vi "Measurement.Free.Initialize.vi"(8 "error in (no error)":errorcluster, 9 "timeout (5000 ms)":i32=5000, 11 "Measurement.Free in":refnum<class "Measurement.Free.lvclass">) -> (0 "error out":errorcluster, 1 "Init complete":bool, 3 "Measurement.Free out":refnum<class "Measurement.Free.lvclass">)   [LabVIEW 2017, in "Measurement.Free.lvclass"]
uses:
  Measurement.Free.lvclass
  SMU/SMU.lvclass
  D:/upwork/Laser Measurement Tool/Laser/project/Subsystems/Device/Device.lvclass
  Device/Device.lvclass
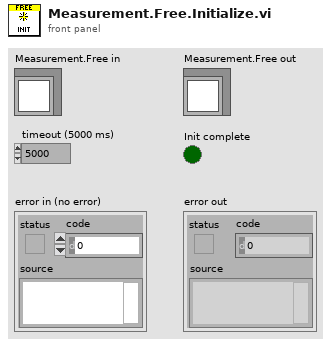
[diagram p1: front panel]
types:
  T1 = typedef "Measurement.Free.lvclass/Configuration--Cluster.ctl" = cluster{"Measurement.Type":enum16{"Free", "I/V Curve", "Wavelength sweeping", "Photocurrent mapping"}, "Configuration.Hardware":T2}
  T2 = typedef "Measurement.Free.lvclass/Configuration.Hardware--Cluster.ctl" = cluster{"Configuration.SMU":T3, "Configuration.LIA":T5, "Configuration.OPM":T7, "Configuration.OPA":T9}
  T3 = typedef "Measurement.Free.lvclass/Configuration.SMU--Cluster.ctl" = cluster{"SMU Model":string, "Configuration":T4}
  T4 = typedef "SMU.lvclass/Configuration--Cluster.ctl" = cluster{"VISA Resource":string, "Channel":string}
  T5 = typedef "Measurement.Free.lvclass/Configuration.LIA--Cluster.ctl" = cluster{"LIA Model":string, "Configuration":T6}
  T6 = typedef "LIA.lvclass/Configuration--Cluster.ctl" = cluster{"VISA Resource":string}
  T7 = typedef "Measurement.Free.lvclass/Configuration.OPM--Cluster.ctl" = cluster{"OPM Model":string, "Configuration":T8}
  T8 = typedef "OPM.lvclass/Configuration--Cluster.ctl" = cluster{"VISA Resource":string}
  T9 = typedef "Measurement.Free.lvclass/Configuration.OPA--Cluster.ctl" = cluster{"OPA Model":string, "Configuration":T10}
  T10 = typedef "OPA.lvclass/Configuration--Cluster.ctl" = cluster{"Serial Number":string}
  T11 = typedef "Measurement.Free.lvclass/Dependencies--Cluster.ctl" = cluster{"SMU":refnum<class "SMU.lvclass">, "LIA":refnum<class "LIA.lvclass">, "OPM":refnum<class "OPM.lvclass">, "OPA":refnum<class "OPA.lvclass">}
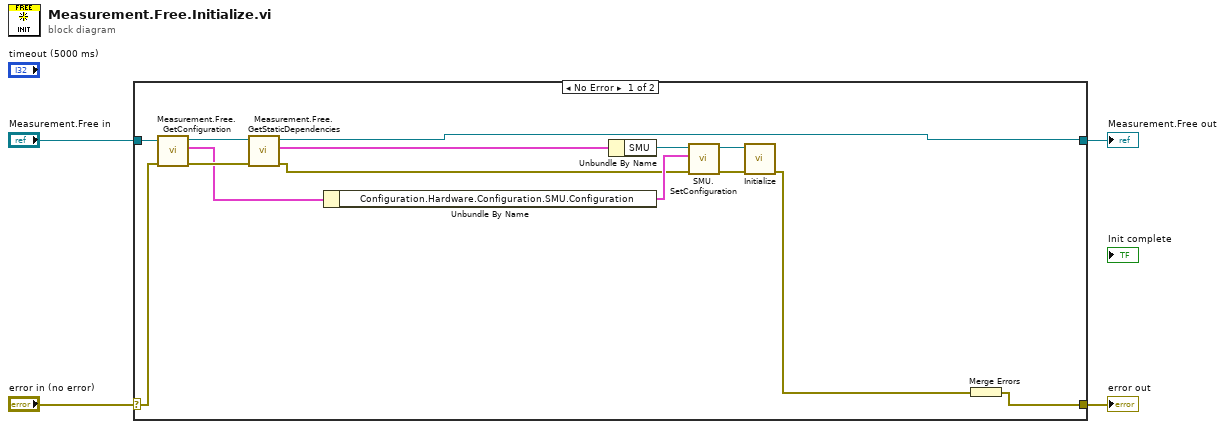
[diagram p0: block diagram]
diagram:
  n1 = case shown="No Error" "error in (no error)" {
    selector: "error in (no error)" -> [w15 w20]
    tunnel: [w5 w20] -> w3
    tunnel: [w8 w19] -> w1
    tunnel: "Measurement.Free in" -> [w17 w19]
    frame No Error {
      n2 = call "Measurement.Free.GetConfiguration.vi"("error in (no error)"=w15, "Measurement.Free"=w17) -> ("error out"=w14:errorcluster, "Configuration"=w13:T1, "Measurement.Free out"=w16:refnum<class "Measurement.Free.lvclass">)  [unwired: 7 in]
      n3 = call "Measurement.Free.GetStaticDependencies.vi"("error in (no error)"=w14, "Measurement.Free"=w16) -> ("error out"=w7:errorcluster, "Dependencies"=w18:T11, "Measurement.Free out"=w8:refnum<class "Measurement.Free.lvclass">)  [unwired: 7 in]
      n4 = Unbundle By Name(w13) -> ("Configuration.Hardware.Configuration.SMU.Configuration"=w11:T4)
      n5 = Unbundle By Name(w18) -> ("SMU"=w12:refnum<class "SMU.lvclass">)
      n6 = call "SMU.SetConfiguration.vi"("error in (no error)"=w7, "Configuration"=w11, "SMU"=w12) -> ("error out"=w9:errorcluster, "SMU out"=w10:refnum<class "SMU.lvclass">)  [unwired: 7 in]
      n7 = call "Initialize.vi"("error in (no error)"=w9, "Device in"=w10) -> ("error out"=w6:errorcluster)  [unwired: 8 in, 1 out]
      n8 = Merge Errors(w6) -> (w5:errorcluster)
    }
    frame Error {
    }
  }
  "error out" <- w3
  "Measurement.Free out" <- w1
